vi "Handle Command.vi"(8 "error in (no error)":errorcluster, 9 "Value":bool, 11 "LatchedValve in":refnum<class "LatchedValve.lvclass">) -> (0 "error out":errorcluster, 3 "LatchedValve out":refnum<class "LatchedValve.lvclass">)   [LabVIEW 2020, in "VolatusControl.lvlib" / "LatchedValve.lvclass"]
uses:
  LatchedValve.lvclass
  LatchedValve.lvclass/LatchedValve.ctl
  State.ctl
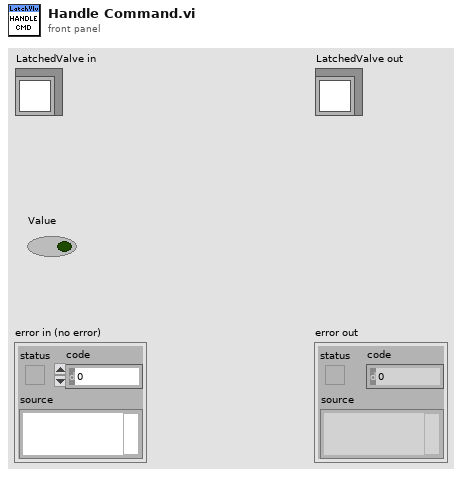
[diagram p1: front panel]
types:
  T1 = typedef "VolatusControl.lvlib/LatchedValve.lvclass/State.ctl" = enum16{"Idle", "Cmd Dir", "Settle Dir", "Cmd En", "Actuate", "Deactivate"}
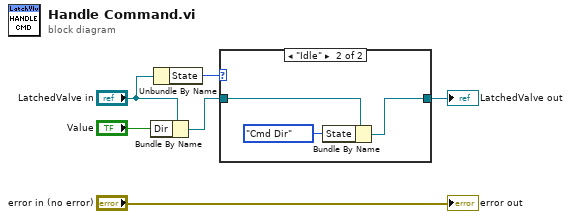
[diagram p0: block diagram]
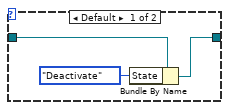
[diagram p2: hidden frame]
diagram:
  n1 = Bundle By Name(cluster="LatchedValve in", "Dir"="Value") -> (w4:refnum<class "LatchedValve.lvclass">)
  n2 = Unbundle By Name("LatchedValve in") -> ("State"=w6:T1)
  n3 = case shown="\"Idle\"" w6 {
    tunnel: w4 -> [w9 w12]
    tunnel: [w7 w10] -> w2
    frame Default {
      n4 = Bundle By Name(cluster=w9, "State"=State."Deactivate") -> (w7:refnum<class "LatchedValve.lvclass">)
    }
    frame "Idle" {
      n5 = Bundle By Name(cluster=w12, "State"=State."Cmd Dir") -> (w10:refnum<class "LatchedValve.lvclass">)
    }
  }
  "LatchedValve out" <- w2
  "error out" <- "error in (no error)"
